vi "Get Date_Heure.vi"() -> (3 "Date_Heure":string)   [LabVIEW 2021]
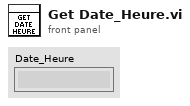
[diagram p1: front panel]
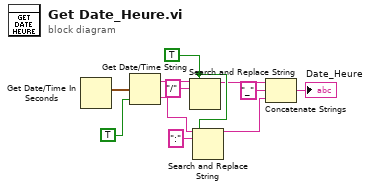
[diagram p0: block diagram]
diagram:
  w10 = TRUE ("tout remplacer ? (F)")
  n1 = Get Date/Time In Seconds() -> (seconds since 1Jan1904=w1:timestamp)
  n2 = Get Date/Time String(seconds (now)=w1, want seconds? (F)=TRUE ("secondes ? (F)")) -> (date string=w3:string, time string=w6:string)  [unwired: 1 in]
  n3 = Search and Replace String(replace all?=w10, input string=w3, search string="/" ("chaîne recherchée")) -> (result string=w7:string)  [unwired: 5 in, 3 out]
  n4 = Search and Replace String(replace all?=w10, input string=w6, search string=":" ("chaîne recherchée")) -> (result string=w9:string)  [unwired: 5 in, 3 out]
  n5 = Concatenate Strings(w7, "_" ("chaîne"), w9) -> (→"Date_Heure":string)
